vi "Read.vi"(0 "I/O In":T1, 9 "Timeout":i32) -> (8 "Data":u8, 14 "# of Elements to Read":u32, 15 "Timed Out?":bool)   [LabVIEW 2012, in "UART 8N1 (FPGA).lvlib"]
uses:
  UART 8N1 (FPGA).lvlib
  <vilib>/rvi/Emulation/niFpgaSctlEmulationGetInTimedLoop.vi
  <vilib>/rvi/DataTransferAndStorage/Container/Common/niFpgaContainerExecOnDevCompGetState.vi
  <vilib>/rvi/DataTransferAndStorage/Container/Common/niFpgaContainerGetUniqueNameForEmu.vi
  <vilib>/rvi/FIFO/Fifo_Resource/nirvififoEmulationSetSize.vi
  <vilib>/rvi/interface/RandomDataEmulation/niFpgaRandomDataHandleErrors.vi
  <vilib>/rvi/interface/RandomDataEmulation/nirviRandomDataFPGAFIFO.vi
  <vilib>/rvi/eio/common/nirviEmuReportErrorAndStop.vi
  <vilib>/rvi/Emulation/niFpgaSctlEmulationFifoFullMgr.vi
  <vilib>/rvi/errors/niFpgaSetErrorForExecOnDevCompSimple.vi
  <vilib>/rvi/DataTransferAndStorage/Container/XNode/niFpgaContainer.xnode
  <vilib>/rvi/FIFO/Fifo_Resource/niFpgaFifoEmulationRefIn.vi
panel:
  # "UART Send\nTxD, 8N1"
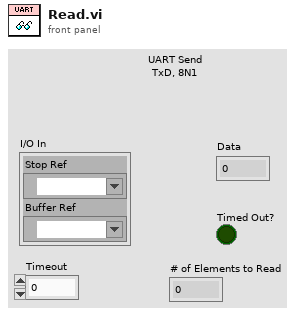
[diagram p1: front panel]
types:
  T1 = cluster{"Stop Ref":refnum<k21>, "Buffer Ref":refnum<k21>}
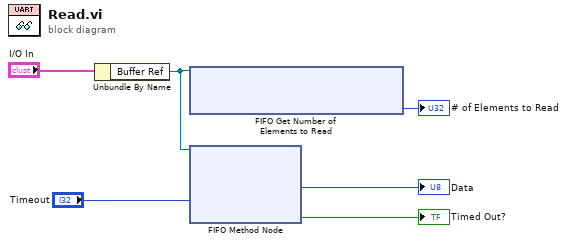
[diagram p0: block diagram]
diagram:
  n1 = Unbundle By Name("I/O In") -> ("Buffer Ref"=w3:refnum<k21>)
  n2 = xnode ("FIFO Get Number of Elements to Read")("FIFO In"=w3) -> ("Number of Elements to Read"=→"# of Elements to Read":u32)  [unwired: 1 out]
  n3 = xnode ("FIFO Method Node")("Timeout"="Timeout", "FIFO In"=w3) -> ("Element"=→"Data":u8, "Timed Out?"=→"Timed Out?":bool)  [unwired: 1 out]
